vi "TMCM351-Init.vi"(2 "错误输入":errorcluster caption="错误输入（无错误）", 3 "Speed /rpm":dbl=50.0 min=0.0 max=2047.0, 4 "com in":refnum<visa-resource-name>) -> (0 "错误输出":errorcluster, 1 "com out":refnum<visa-resource-name>)   [LabVIEW 2018]
uses:
  Device VIs/Verbal.vi
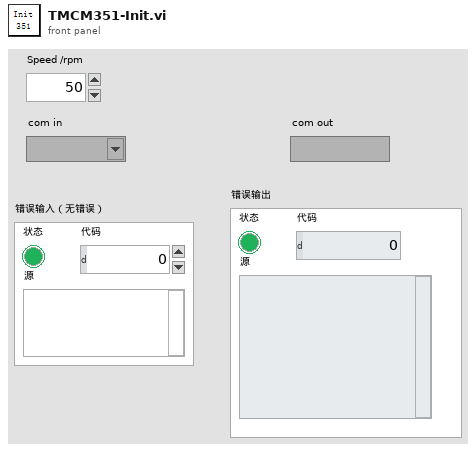
[diagram p1: front panel]
types:
  T1 = enum8{"full", "half", "4", "8", "16", "32", "64"}
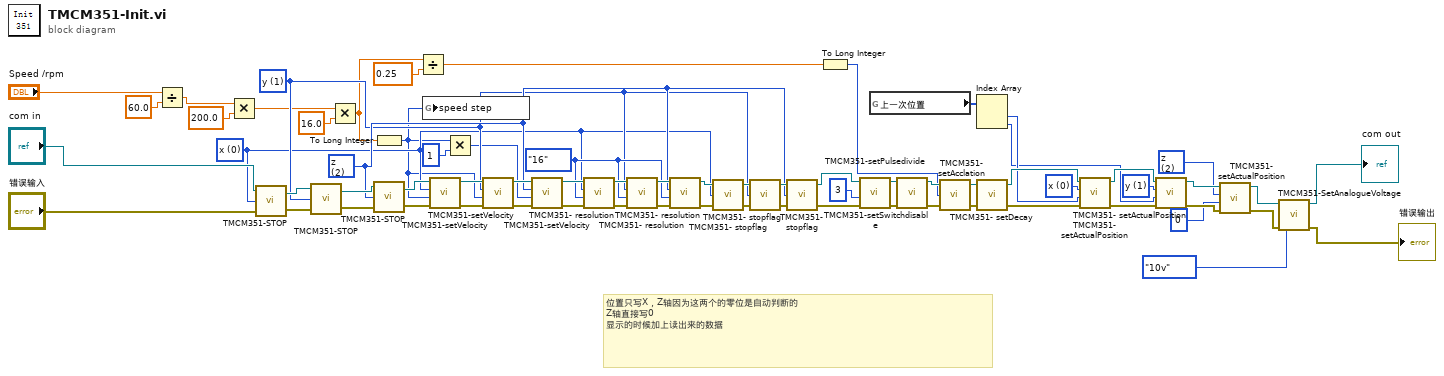
[diagram p0: block diagram]
diagram:
  w7 = u8 2 items=["x", "y", "z"] ("motor")
  w11 = u8 1 items=["x", "y", "z"] ("motor")
  w16 = u8 0 items=["x", "y", "z"] ("motor")
  w50 = T1."16" ("reasulotion")
  w43 = u8 2 items=["x", "y", "z"] ("motor")
  w42 = u8 1 items=["x", "y", "z"] ("motor")
  w41 = u8 0 items=["x", "y", "z"] ("motor")
  # "位置只写X，Z轴因为这两个的零位是自动判断的\nZ轴直接写0\n显示的时候加上读出来的数据"
  n1 = Divide(x="Speed /rpm", y=60.0) -> (x/y=w33:dbl)
  n2 = Multiply(x=w33, y=200.0) -> (x*y=w31:dbl)
  n3 = call "TMCM351-STOP.vi"("错误输入"="错误输入", "motor"=w41, "com in"="com in") -> ("错误输出"=w66:errorcluster, "com out"=w67:refnum<visa-resource-name>)
  n4 = call "TMCM351-STOP.vi"("错误输入"=w66, "motor"=w42, "com in"=w67) -> ("错误输出"=w64:errorcluster, "com out"=w65:refnum<visa-resource-name>)
  n5 = Multiply(x=w31, y=16.0) -> (x*y=w29:dbl)
  n6 = To Long Integer(number=w29) -> (32bit integer=w23:i32)
  n7 = call "TMCM351-STOP.vi"("错误输入"=w64, "motor"=w43, "com in"=w65) -> ("错误输出"=w62:errorcluster, "com out"=w63:refnum<visa-resource-name>)
  n8 = Divide(x=w29, y=0.25) -> (x/y=w27:dbl)
  n9 = global write "Verbal.vi" "speed step"(w23) -> ()
  n10 = call "TMCM351-setVelocity.vi"("错误输入"=w62, "Speed"=w23, "motor"=w41, "com in"=w63) -> ("错误输出"=w61:errorcluster, "com out"=w60:refnum<visa-resource-name>)  [unwired: 2 in]
  n11 = Multiply(x=w23, y=1) -> (x*y=w21:i32)
  n12 = call "TMCM351-setVelocity.vi"("错误输入"=w61, "Speed"=w23, "motor"=w42, "com in"=w60) -> ("错误输出"=w59:errorcluster, "com out"=w58:refnum<visa-resource-name>)  [unwired: 2 in]
  n13 = call "TMCM351-setVelocity.vi"("错误输入"=w59, "Speed"=w21, "motor"=w43, "com in"=w58) -> ("错误输出"=w55:errorcluster, "com out"=w56:refnum<visa-resource-name>)  [unwired: 2 in]
  n14 = call "TMCM351- resolution.vi"("错误输入"=w55, "reasulotion"=w50, "motor"=w41, "com in"=w56) -> ("错误输出"=w54:errorcluster, "com out"=w53:refnum<visa-resource-name>)  [unwired: 2 in]
  n15 = call "TMCM351- resolution.vi"("错误输入"=w54, "reasulotion"=w50, "motor"=w42, "com in"=w53) -> ("错误输出"=w52:errorcluster, "com out"=w51:refnum<visa-resource-name>)  [unwired: 2 in]
  n16 = call "TMCM351- resolution.vi"("错误输入"=w52, "reasulotion"=w50, "motor"=w43, "com in"=w51) -> ("错误输出"=w48:errorcluster, "com out"=w49:refnum<visa-resource-name>)  [unwired: 2 in]
  n17 = call "TMCM351- stopflag.vi"("错误输入"=w48, "motor"=w41, "com in"=w49) -> ("错误输出"=w47:errorcluster, "com out"=w46:refnum<visa-resource-name>)  [unwired: 1 in]
  n18 = call "TMCM351- stopflag.vi"("错误输入"=w47, "motor"=w42, "com in"=w46) -> ("错误输出"=w44:errorcluster, "com out"=w45:refnum<visa-resource-name>)  [unwired: 1 in]
  n19 = call "TMCM351- stopflag.vi"("错误输入"=w44, "motor"=w43, "com in"=w45) -> ("错误输出"=w39:errorcluster, "com out"=w40:refnum<visa-resource-name>)  [unwired: 1 in]
  n20 = To Long Integer(number=w27) -> (32bit integer=w24:i32)
  n21 = call "TMCM351-setPulsedivide.vi"("错误输入"=w39, "pulse_divid"=3, "com in"=w40) -> ("错误输出"=w36:errorcluster, "com out"=w37:refnum<visa-resource-name>)  [unwired: 3 in]
  n22 = global read "Verbal.vi" "上一次位置"() -> (w18:i32[])
  n23 = call "TMCM351-setSwitchdisable.vi"("错误输入"=w36, "com in"=w37) -> ("错误输出"=w25:errorcluster, "com out"=w26:refnum<visa-resource-name>)  [unwired: 4 in]
  n24 = call "TMCM351- setAcclation.vi"("错误输入"=w25, "Acclation"=w24, "com in"=w26) -> ("错误输出"=w19:errorcluster, "com out"=w20:refnum<visa-resource-name>)  [unwired: 1 in]
  n25 = Index Array(array=w18) -> (element #1=w15:i32, element #2=w10:i32)  [unwired: 2 in]
  n26 = call "TMCM351- setDecay.vi"("错误输入"=w19, "com in"=w20) -> ("错误输出"=w14:errorcluster, "com out"=w17:refnum<visa-resource-name>)  [unwired: 2 in]
  n27 = call "TMCM351- setActualPosition.vi"("错误输入"=w14, "Position"=w15, "motor"=w16, "com in"=w17) -> ("错误输出"=w12:errorcluster, "com out"=w13:refnum<visa-resource-name>)  [unwired: 2 in]
  n28 = call "TMCM351- setActualPosition.vi"("错误输入"=w12, "Position"=w10, "motor"=w11, "com in"=w13) -> ("错误输出"=w8:errorcluster, "com out"=w9:refnum<visa-resource-name>)  [unwired: 2 in]
  n29 = call "TMCM351- setActualPosition.vi"("错误输入"=w8, "Position"=0, "motor"=w7, "com in"=w9) -> ("错误输出"=w2:errorcluster, "com out"=w5:refnum<visa-resource-name>)  [unwired: 2 in]
  n30 = call "TMCM351-SetAnalogueVoltage.vi"("错误输入"=w2, "数据"=enum16{"3.3v", "10v"}."10v", "com in"=w5) -> ("错误输出"=→"错误输出":errorcluster, "com out"=→"com out":refnum<visa-resource-name>)  [unwired: 2 in, 1 out]
